vi "HelioScan_3.vi"() -> ()   [LabVIEW 2010]
uses:
  labview_source/controls/update_picture.ctl
  common/xcontrols/XUserDropdown/XUserDropdown/XUserDropdown.xctl
  tools/HelioUpdateMH100803/HelioUpdateMH100803/HelioUpdateMH100803.lvclass
  common/classes/ErrorController/ErrorController/ErrorController.lvclass
  labview_source/type_definitions/clusters/controls_refs.ctl
  components/DAQ/GenericDAQ/GenericDAQ/GenericDAQ.lvclass
  components/ImageAssembler/GenericImageAssembler/GenericImageAssembler/GenericImageAssembler.lvclass
  components/DataCollection/GenericDataCollection/GenericDataCollection/GenericDataCollection.lvclass
  components/Display/GenericDisplay/GenericDisplay/GenericDisplay.lvclass
  components/Analyser/GenericAnalyser/GenericAnalyser/GenericAnalyser.lvclass
  components/ImagingMode/GenericImagingMode/GenericImagingMode/GenericImagingMode.lvclass
  components/Instrument/GenericInstrument/GenericInstrument/GenericInstrument.lvclass
  components/ScanHead/GenericScanHead/GenericScanHead/GenericScanHead.lvclass
  components/Stimulator/GenericStimulator/GenericStimulator/GenericStimulator.lvclass
  components/ExperimentController/GenericExperimentController/GenericExperimentController/GenericExperimentController.lvclass
  components/Stage/GenericStage/GenericStage/GenericStage.lvclass
  <vilib>/Utility/miscctls.llb/LVPointTypeDef.ctl
  components/DataCollection/GenericDataCollection/GenericDataCollection/trigger_enum.ctl
  common/classes/GenericComponent/GenericComponent/GenericComponent.lvclass
  <vilib>/Platform/browser.llb/Open URL in Default Browser (string).vi
  common/classes/ErrorController/ErrorController/class_data.vi
panel:
  out "saving message":string
  out "progress slider":u8(slide) caption="slider" scale=0.0..11.0
  in  "button:start_experiment":bool
  in  "button:start_single_sweep":bool
  in  "button:start_focus":bool
  in  "user":string(xcontrol)
  out "update icon":T1
  in  "file base name":string
  in  "data folder path":path
  in  "notebook":string caption="Notebook"
  in  "exit_button":bool
  in  "objective":string(combo)
  in  "save button":bool
  in  "settings tab":T2(tab)
  in  "imaging mode":string(combo)
  in  "experimental protocol":string(combo)
  in  "stimulator enabled?":bool
  in  "button: task manager":bool
  out "error handler":bool caption="error controller"
  out "experiment controller":bool
  out "imaging mode":bool
  out "scan head":bool
  out "DAQ":bool
  out "image assembler":bool
  out "data collection":bool
  out "display":bool
  out "analyser":bool
  out "stage":bool
  out "stimulator":bool
  out "instrument":bool
  out "Message":string="No Error"
  in  "title":bool caption="HelioScan 3.10.0"
  # "Note: stimulator only works in \"single sweep mode\" and \"experiment mode\"!"
  # "Loaded"
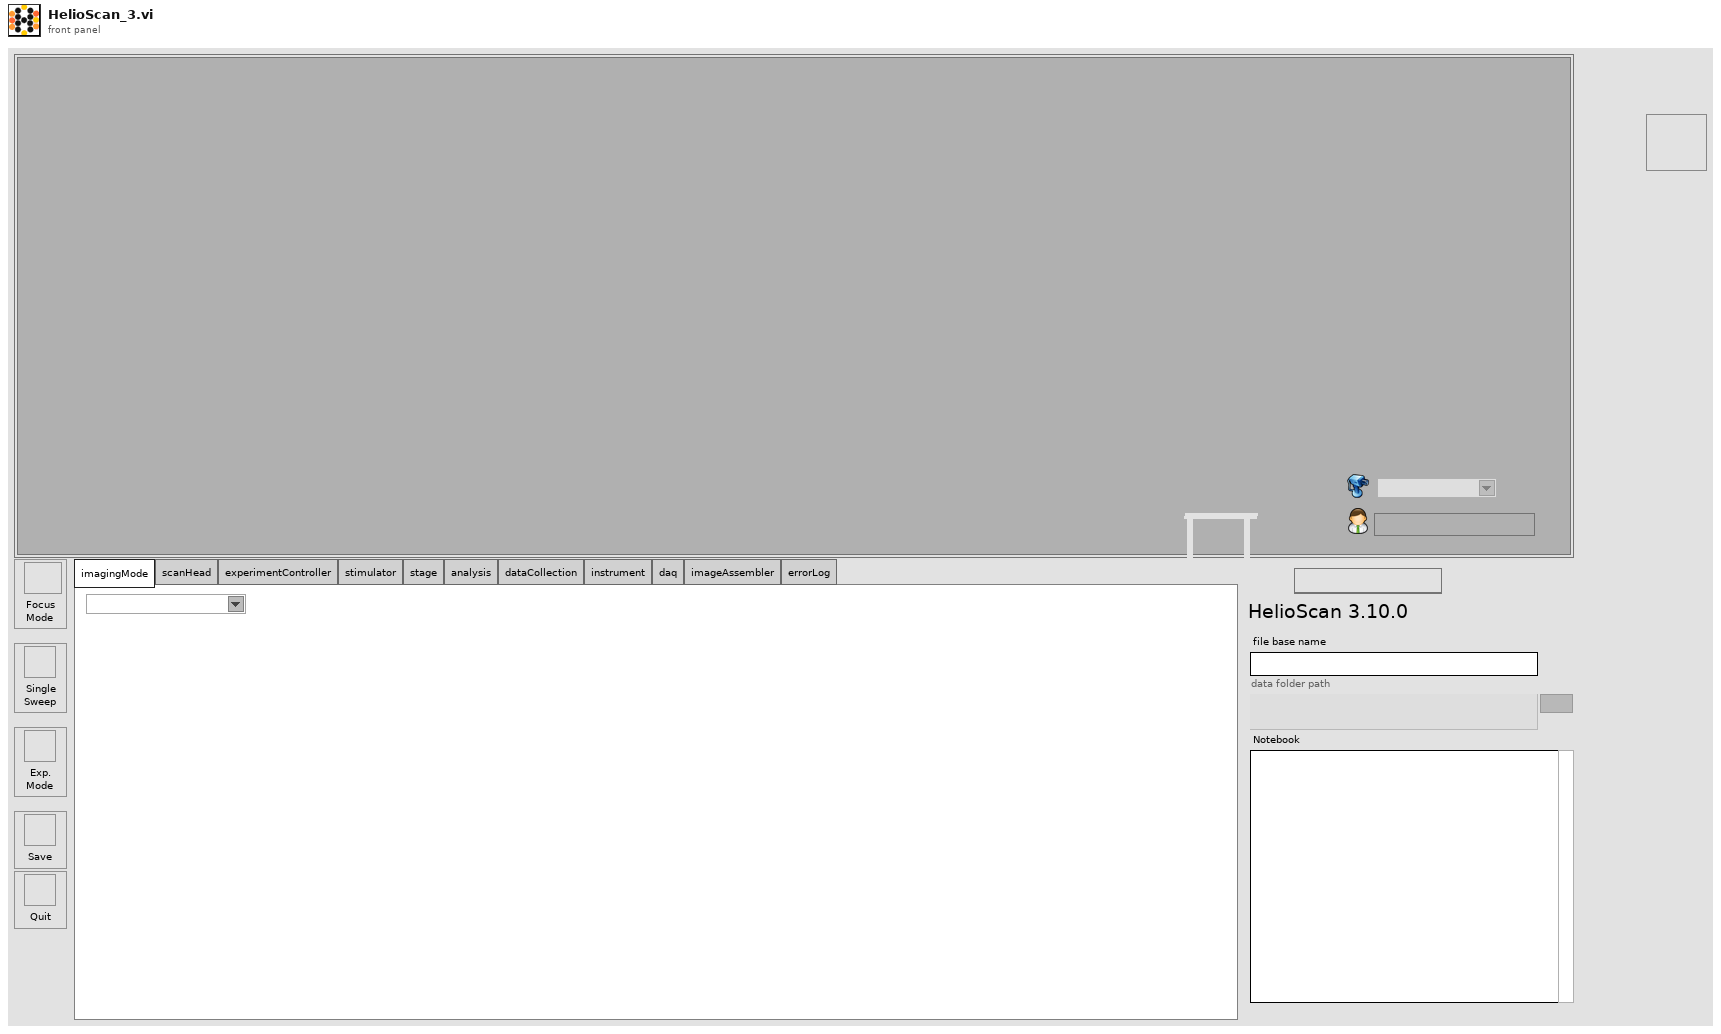
[diagram p1: front panel]
types:
  T1 = typedef "HelioUpdateMH100803.lvclass/update_picture.ctl" = u16
  T2 = enum32{"imagingMode", "scanHead", "experimentController", "stimulator", "stage", "analysis", "dataCollection", "instrument", "daq", "imageAssembler", "errorLog"}
  T3 = typedef "controls_refs.ctl" = cluster{"buttons":cluster{"start_focus":refnum<vi>, "start_single_sweep":refnum<vi>, "start_experiment":refnum<vi>, "save":refnum<vi>, "exit":refnum<vi>}, "tabs":cluster{"main":refnum<vi>, "settings":refnum<vi>}, "subpanels":cluster{"imagingMode":refnum<vi>, "scanHead":refnum<vi>, "display":refnum<vi>, "experimentController":refnum<vi>, "instrument":refnum<vi>, "stage":refnum<vi>, "stimulator":refnum<vi>, "dataCollection":refnum<vi>, "analyser":refnum<vi>, "daq":refnum<vi>, "imageAssembler":refnum<vi>}, "drop-downs":cluster{"imagingMode":refnum<vi>, "experimentalController":refnum<vi>, "objective":refnum<vi>}, "status lights":cluster{"experimentController":refnum<vi>, "imagingMode":refnum<vi>, "scanHead":refnum<vi>, "daq":refnum<vi>, "imageAssembler":refnum<vi>, "dataCollection":refnum<vi>, "display":refnum<vi>, "analyser":refnum<vi>, "stage":refnum<vi>, "stimulator":refnum<vi>, "instrument":refnum<vi>}, "message":refnum<vi>, "stimulator enabled?":refnum<vi>, "saving":cluster{"data folder path":refnum<vi>, "file base name":refnum<vi>, "notebook":refnum<vi>}, "progress bar":refnum<vi>, "update icon":refnum<vi>, "title":refnum<vi>, "main vi":refnum<vi>, "user":refnum<vi>}
  T4 = typedef "LVPointTypeDef.ctl" = cluster{"Horizontal":i16, "Vertical":i16}
  T5 = typedef "GenericDataCollection.lvclass/trigger_enum.ctl" = enum16{"NULL", "save", "reset"}
  T6 = enum32{"Invalid", "Standard", "Closed", "Hidden", "Minimized", "Maximized"}
  T7 = enum8{"Enabled", "Disabled", "Disabled and Grayed Out"}
  T8 = enum16{"focus mode", "single sweep mode", "experiment mode"}
  T9 = typedef "main_trigger_enum.ctl" = enum16{"NULL", "initialise", "terminate", "start", "stop", "change objective", "change experimentController", "change imagingMode", "save notebook", "started saving", "finished saving", "expCtr ready", "expCtr missing", "imgMd ready", "imgMd missing", "scanHd ready", "scanHd missing", "DAQ ready", "DAQ missing", "imgAsm ready", "imgAsm missing", "dataColl ready", "dataColl missing", "display ready", "display missing", "analysr ready", "analysr missing", "instrmnt ready", "instrmnt missing", "stimltr ready", "stimltr missing", "stage ready", "stage missing"}
  T10 = typedef "run_mode_enum.ctl" = enum16{"focus mode", "single sweep mode", "experiment mode"}
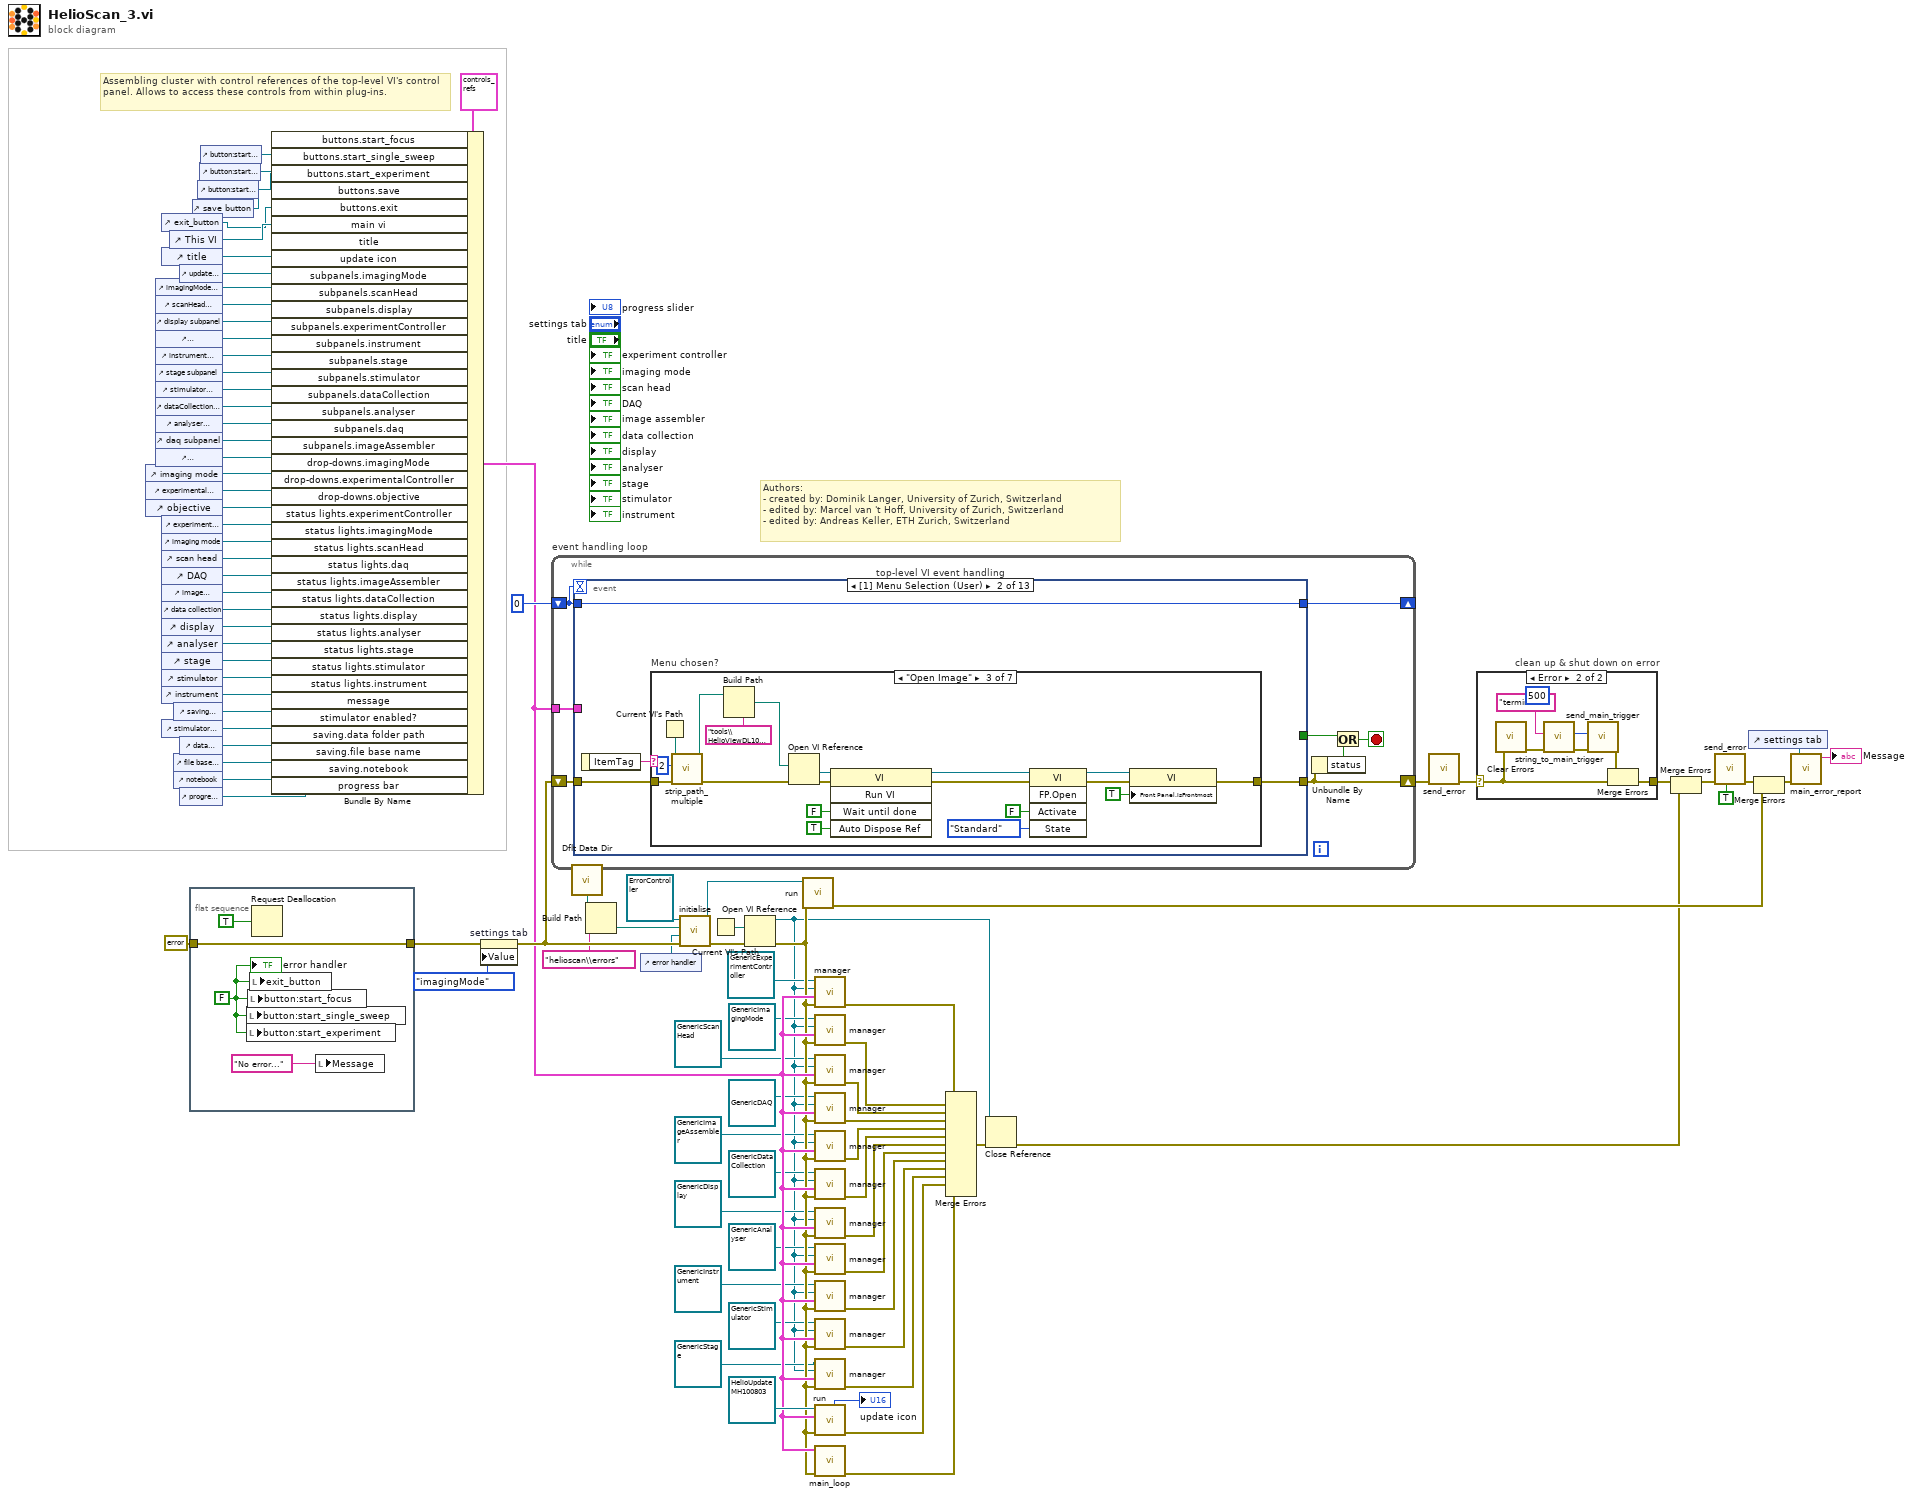
[diagram p0: block diagram]
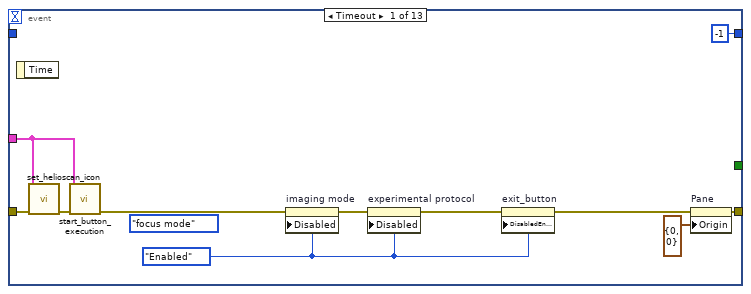
[diagram p3: hidden frame]
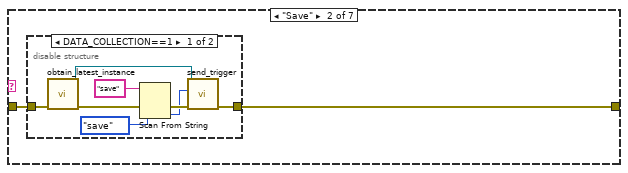
[diagram p5: hidden frame]
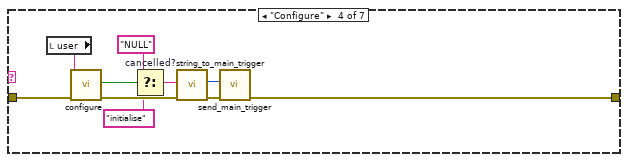
[diagram p7: hidden frame]
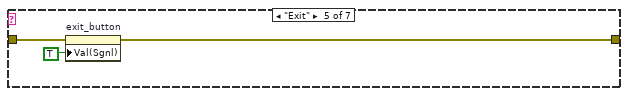
[diagram p8: hidden frame]
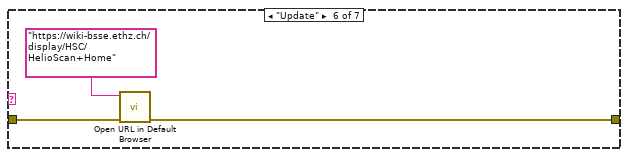
[diagram p9: hidden frame]
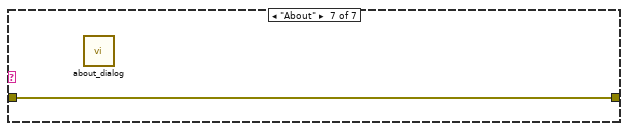
[diagram p10: hidden frame]
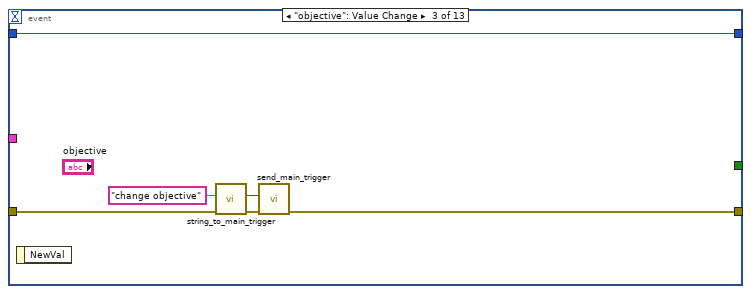
[diagram p11: hidden frame]
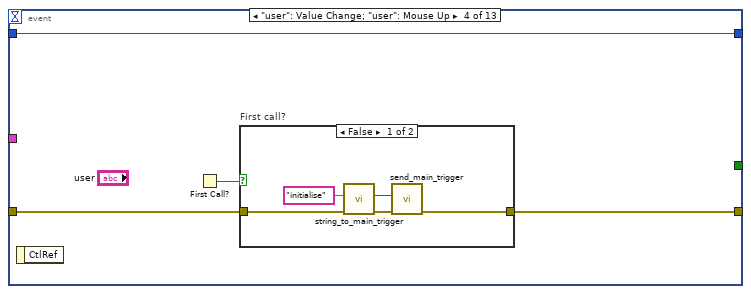
[diagram p12: hidden frame]
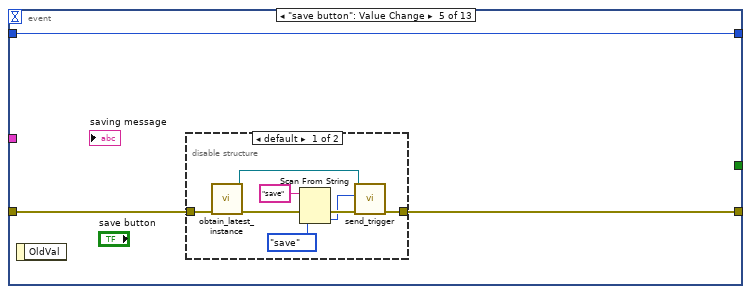
[diagram p14: hidden frame]
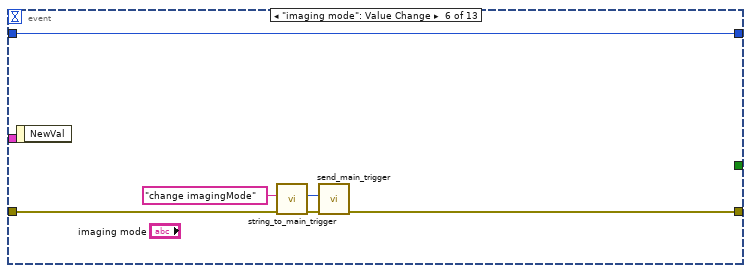
[diagram p16: hidden frame]
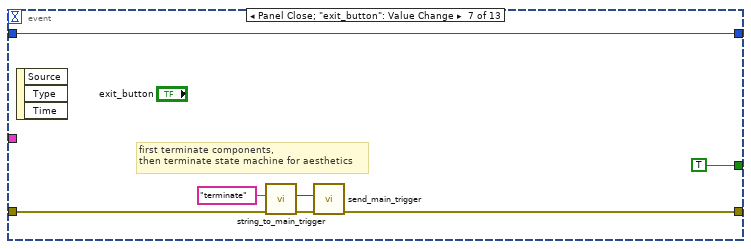
[diagram p17: hidden frame]
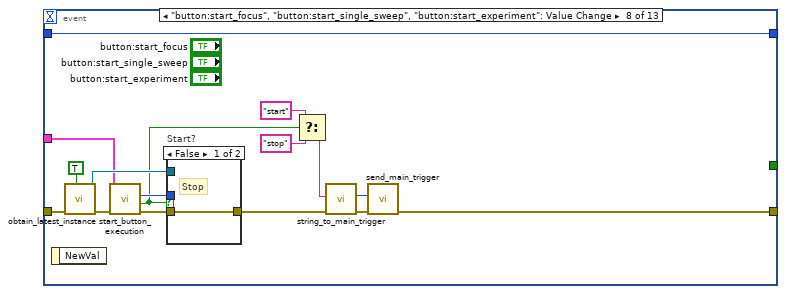
[diagram p18: hidden frame]
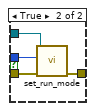
[diagram p19: hidden frame]
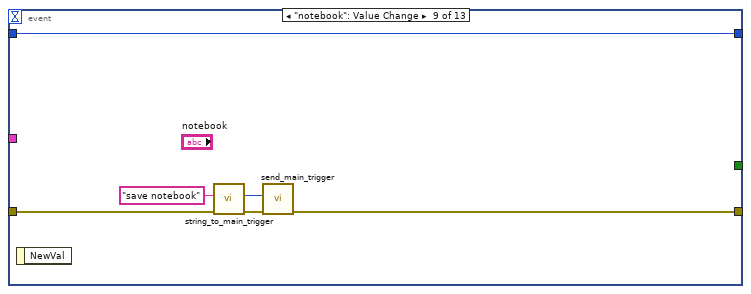
[diagram p20: hidden frame]
diagram:
  # "Authors: \n- created by: Dominik Langer, University of Zurich, Switzerland\n- edited by: Marcel van 't Hoff, University of Zurich, Switzerland\n- edited by: Andreas Keller, ETH Zurich, Switzerland"
  # "Assembling cluster with control references of the top-level VI's control panel. Allows to access these controls from within plug-ins."
  n1 = control-ref of="imaging mode"() -> (w83:refnum<vi>)
  n2 = control-ref of="experimental protocol"() -> (w84:refnum<vi>)
  n3 = control-ref of="objective"() -> (w69:refnum<vi>)
  n4 = control-ref of="imagingMode subpanel"() -> (w63:refnum<vi>)
  n5 = control-ref of="scanHead subpanel"() -> (w94:refnum<vi>)
  n6 = control-ref of="display subpanel"() -> (w90:refnum<vi>)
  n7 = control-ref of="experimentController subpanel"() -> (w91:refnum<vi>)
  n8 = control-ref of="instrument subpanel"() -> (w89:refnum<vi>)
  n9 = control-ref of="stage subpanel"() -> (w87:refnum<vi>)
  n10 = control-ref of="stimulator subpanel"() -> (w86:refnum<vi>)
  n11 = control-ref of="dataCollection subpanel"() -> (w85:refnum<vi>)
  n12 = control-ref of="analyser subpanel"() -> (w82:refnum<vi>)
  n13 = control-ref of="daq subpanel"() -> (w61:refnum<vi>)
  n14 = control-ref of="imageAssembler subpanel"() -> (w62:refnum<vi>)
  n15 = control-ref of="exit_button"() -> (w1:refnum<vi>)
  n16 = control-ref of="title"() -> (w44:refnum<vi>)
  n17 = control-ref of="experiment controller"() -> (w73:refnum<vi>)
  n18 = control-ref of="imaging mode"() -> (w72:refnum<vi>)
  n19 = control-ref of="scan head"() -> (w76:refnum<vi>)
  n20 = control-ref of="DAQ"() -> (w75:refnum<vi>)
  n21 = control-ref of="image assembler"() -> (w74:refnum<vi>)
  n22 = control-ref of="data collection"() -> (w71:refnum<vi>)
  n23 = control-ref of="display"() -> (w77:refnum<vi>)
  n24 = control-ref of="analyser"() -> (w78:refnum<vi>)
  n25 = control-ref of="stage"() -> (w81:refnum<vi>)
  n26 = control-ref of="stimulator"() -> (w80:refnum<vi>)
  n27 = control-ref of="instrument"() -> (w70:refnum<vi>)
  n28 = control-ref of="stimulator enabled?"() -> (w67:refnum<vi>)
  n29 = control-ref of="This VI"() -> (w41:refnum<vi>)
  n30 = control-ref of="saving message"() -> (w45:refnum<vi>)
  n31 = control-ref of="file base name"() -> (w65:refnum<vi>)
  n32 = control-ref of="notebook"() -> (w64:refnum<vi>)
  n33 = control-ref of="update icon"() -> (w43:refnum<vi>)
  n34 = control-ref of="data folder path"() -> (w66:refnum<vi>)
  n35 = control-ref of="progress bar"() -> (w49:refnum<vi>)
  n36 = flat-sequence {
    tunnel: errorcluster {"status"=FALSE, "code"=0, "source"=""} ("error in (no error)") -> [w98]
    tunnel: [w98] -> w7
    frame #0 {
      w95 = FALSE
      n37 = local write "button:start_single_sweep"(w95) -> ()
      n38 = local write "button:start_experiment"(w95) -> ()
      n39 = local write "button:start_focus"(w95) -> ()
      n40 = local write "exit_button"(w95) -> ()
      n41 = Request Deallocation(TRUE ("flag")) -> ()
      n42 = local write "Message"("No error...") -> ()
      "error handler" <- w95
    }
  }
  n43 = control-ref of="save button"() -> (w2:refnum<vi>)
  n44 = control-ref of="button:start_experiment"() -> (w3:refnum<vi>)
  n45 = control-ref of="button:start_single_sweep"() -> (w4:refnum<vi>)
  n46 = control-ref of="button:start_focus"() -> (w5:refnum<vi>)
  n47 = Bundle By Name(cluster=T3 {"buttons"={"start_focus"=refnum, "start_single_sweep"=refnum, "start_experiment"=refnum, "save"=refnum, "exit"=refnum}, "tabs"={"main"=refnum, "settings"=refnum}, "subpanels"={"imagingMode"=refnum, "scanHead"=refnum, "display"=refnum, "experimentController"=refnum, "instrument"=refnum, "stage"=refnum, "stimulator"=refnum, "dataCollection"=refnum, "analyser"=refnum, "daq"=refnum, "imageAssembler"=refnum}, "drop-downs"={"imagingMode"=refnum, "experimentalController"=refnum, "objective"=refnum}, "status lights"={"experimentController"=refnum, "imagingMode"=refnum, "scanHead"=refnum, "daq"=refnum, "imageAssembler"=refnum, "dataCollection"=refnum, "display"=refnum, "analyser"=refnum, "stage"=refnum, "stimulator"=refnum, "instrument"=refnum}, "message"=refnum, "stimulator enabled?"=refnum, "saving"={"data folder path"=refnum, "file base name"=refnum, "notebook"=refnum}, "progress bar"=refnum, "update icon"=refnum, "title"=refnum, "main vi"=refnum, "user"=refnum} ("control references"), "buttons.start_focus"=w5, "buttons.start_single_sweep"=w4, "buttons.start_experiment"=w3, "buttons.save"=w2, "buttons.exit"=w1, "main vi"=w41, "title"=w44, "update icon"=w43, "subpanels.imagingMode"=w63, "subpanels.scanHead"=w94, "subpanels.display"=w90, "subpanels.experimentController"=w91, "subpanels.instrument"=w89, "subpanels.stage"=w87, "subpanels.stimulator"=w86, "subpanels.dataCollection"=w85, "subpanels.analyser"=w82, "subpanels.daq"=w61, "subpanels.imageAssembler"=w62, "drop-downs.imagingMode"=w83, "drop-downs.experimentalController"=w84, "drop-downs.objective"=w69, "status lights.experimentController"=w73, "status lights.imagingMode"=w72, "status lights.scanHead"=w76, "status lights.daq"=w75, "status lights.imageAssembler"=w74, "status lights.dataCollection"=w71, "status lights.display"=w77, "status lights.analyser"=w78, "status lights.stage"=w81, "status lights.stimulator"=w80, "status lights.instrument"=w70, "message"=w45, "stimulator enabled?"=w67, "saving.data folder path"=w66, "saving.file base name"=w65, "saving.notebook"=w64, "progress bar"=w49) -> (w23:T3)
  n48 = property on="settings tab" class="TabCtl (strict)"(error in=w7, "Value"=T2."imagingMode" ("settings tab")) -> (error out=w35:errorcluster)  [unwired: 1 in, 1 out]
  n49 = while "event handling loop" {
    shift-right: [w104] -> _
    shift-left: 0 -> [w105]
    tunnel: w23 -> [w103]
    shift-right: [w102] -> w38
    shift-left: w35 -> [w106]
    stop <- w99 stop-if-true
    n50 = event "top-level VI event handling" shown="[1] Menu Selection (User)" {
      selector: _ -> [_ _ _ _ _ _ _ _ _ _ _ _ _]
      dyn-events: _ -> [_ _ _ _ _ _ _ _ _ _ _ _ _]
      timeout: w105 -> [_ _ _ _ _ _ _ _ _ _ _ _ _]
      tunnel: [_ _ _ _ _ _ TRUE _ _ _ _ _ _] -> w101
      tunnel: [w115 w118 w174 w178 w187 w202 w208 w212 w236 w242 w251 w262 w268] -> w102
      tunnel: w106 -> [w111 w119 w173 w176 w186 w201 w204 w216 w235 w243 w256 w259 w279]
      tunnel: [-1 w121 w175 w179 w188 w203 w210 w226 w237 w245 w257 w263 w280] -> w104
      tunnel: w105 -> [_ w121 w175 w179 w188 w203 w210 w226 w237 w245 w257 w263 w280]
      tunnel: w103 -> [w109 _ _ _ _ _ _ w213 _ _ _ _ _]
      event Timeout {
        w112 = T7."Enabled" ("Disabled")
        (unwired) T8."focus mode" ("Value (Signaling)")
        n51 = event-data() -> ()  [unwired: 2 out]
        n52 = call "set_helioscan_icon.vi"("error in (no error)"=w111, "reference cluster in"=w109) -> ("error out"=w110:errorcluster)  [unwired: 9 in]
        n53 = call "start_button_execution.vi"("error in (no error)"=w110, "control references"=w109) -> ("error out"=w108:errorcluster)  [unwired: 7 in, 2 out]
        n54 = property on="imaging mode" class="CmbBox"(error in=w108, "Disabled"=w112) -> (error out=w116:errorcluster)  [unwired: 1 in, 1 out]
        n55 = property on="experimental protocol" class="CmbBox"(error in=w116, "Disabled"=w112) -> (error out=w113:errorcluster)  [unwired: 1 in, 1 out]
        n56 = property on="exit_button" class="Bool (strict)"(error in=w113, "DisabledEnum"=w112) -> (error out=w107:errorcluster)  [unwired: 1 in, 1 out]
        n57 = property on="Pane" class="Pane"(error in=w107, "Origin"=T4 {"Horizontal"=0, "Vertical"=0}) -> (error out=w115:errorcluster)  [unwired: 1 in, 1 out]
      }
      event Menu Selection (User) {
        n58 = event-data() -> ("ItemTag"=w120:string)  [unwired: 1 out]
        n59 = case "Menu chosen?" shown="\"Open Image\"" w120 {
          tunnel: w119 -> [w122 w124 w149 w162 w165 w168 w169]
          tunnel: [w122 w123 w135 w160 w163 w167 w169] -> w118
          frame Default {
          }
          frame "Save" {
            n60 = disable-structure shown="DATA_COLLECTION==1" {
              disable-tunnel: w124 -> [w131 w133]
              disable-tunnel: [w132 w133] -> w123
              frame condition #0 (active) {
                n61 = call "obtain_latest_instance.vi"("error in (no error)"=w131) -> ("error out"=w128:errorcluster, "GenericDataCollection out"=w130:refnum<class "GenericDataCollection.lvclass">)  [unwired: 1 in, 8 out]
                n62 = Scan From String(input string="save", error in=w128, default 1=trigger_enum."save" ("trigger")) -> (error out=w127:errorcluster, output 1=w126:T5)  [unwired: 2 in, 2 out]
                n63 = call-dynamic "send_trigger.vi"("error in (no error)"=w127, "trigger"=w126, "GenericDataCollection in"=w130) -> ("error out"=w132:errorcluster)  [unwired: 8 out]
              }
              frame condition #1 {
              }
            }
          }
          frame "Open Image" {
            n64 = Current VI's Path() -> (path=w150:path)
            n65 = call "strip_path_multiple.vi"("error in (no error)"=w149, "number of strips"=2, "path in"=w150) -> ("error out"=w148:errorcluster, "path out"=w144:path)  [unwired: 7 in]
            n66 = Build Path(base path=w144, name or relative path="tools\\HelioViewDL100122\\HelioView.vi") -> (appended path=w142:path)
            n67 = Open VI Reference(vi path=w142, error in (no error)=w148) -> (vi reference=w152:refnum<vi>, error out=w151:errorcluster)  [unwired: 4 in]
            n68 = invoke class="VI" method="Run VI"(reference=w152, error in=w151, "Wait until done"=FALSE ("Wait Until Done"), "Auto Dispose Ref"=TRUE ("Auto Dispose Reference")) -> (reference out=w138:refnum<vi>, error out=w141:errorcluster)  [unwired: 1 in, 3 out]
            n69 = invoke class="VI" method="FP.Open"(reference=w138, error in=w141, "Activate"=FALSE ("Activate?"), "State"=T6."Standard") -> (reference out=w134:refnum<vi>, error out=w136:errorcluster)  [unwired: 1 in, 3 out]
            n70 = property class="VI"(reference=w134, error in=w136, "Front Panel.IsFrontmost"=TRUE ("Front Panel Window:Is Frontmost")) -> (error out=w135:errorcluster)  [unwired: 1 out]
          }
          frame "Configure" {
            n71 = local read "user"() -> (w161:string)
            n72 = call "configure.vi"("error in (no error)"=w162, "user"=w161) -> ("error out"=w158:errorcluster, "cancelled?"=w159:bool)  [unwired: 1 in, 7 out]
            n73 = Select "cancelled?"(t="NULL", s=w159, f="initialise") -> (s? t:f=w154:string)
            n74 = call "string_to_main_trigger.vi"("error in (no error)"=w158, "trigger string"=w154) -> ("error out"=w157:errorcluster, "main trigger"=w153:T9)  [unwired: 8 in]
            n75 = call "send_main_trigger.vi"("error in (no error)"=w157, "trigger"=w153) -> ("error out"=w160:errorcluster)  [unwired: 9 in]
          }
          frame "Exit" {
            n76 = property on="exit_button" class="Bool (strict)"(error in=w165, "Val(Sgnl)"=TRUE) -> (error out=w163:errorcluster)  [unwired: 1 in, 1 out]
          }
          frame "Update" {
            n77 = call-poly <vilib>:"Open URL in Default Browser.vi"("error in (no error)"=w168, "URL"="https://wiki-bsse.ethz.ch/display/HSC/HelioScan+Home") -> ("error out"=w167:errorcluster)  [unwired: 4 in, 1 out]
          }
          frame "About" {
            n78 = call "about_dialog.vi"() -> ()  [unwired: 1 out]
          }
        }
      }
      event "objective": Value Change {
        n79 = event-data() -> ()  [unwired: 2 out]
        n80 = call "string_to_main_trigger.vi"("error in (no error)"=w173, "trigger string"="change objective") -> ("error out"=w172:errorcluster, "main trigger"=w171:T9)  [unwired: 8 in]
        n81 = call "send_main_trigger.vi"("error in (no error)"=w172, "trigger"=w171) -> ("error out"=w174:errorcluster)  [unwired: 9 in]
      }
      event "user": Value Change; "user": Mouse Up {
        n82 = event-data() -> ()  [unwired: 2 out]
        n83 = First Call?() -> (First Call?: T/F=w177:bool)
        n84 = case "First call?" shown="False" w177 {
          tunnel: [w184 w185] -> w178
          tunnel: w176 -> [w183 w185]
          frame False {
            n85 = call "string_to_main_trigger.vi"("error in (no error)"=w183, "trigger string"="initialise") -> ("error out"=w182:errorcluster, "main trigger"=w181:T9)  [unwired: 8 in]
            n86 = call "send_main_trigger.vi"("error in (no error)"=w182, "trigger"=w181) -> ("error out"=w184:errorcluster)  [unwired: 9 in]
          }
          frame True {
          }
        }
      }
      event "save button": Value Change {
        n87 = event-data() -> ()  [unwired: 2 out]
        n88 = disable-structure shown="default" {
          disable-tunnel: [w196 w197] -> w187
          disable-tunnel: w186 -> [w195 w197]
          frame condition #0 (active) {
            n89 = call "obtain_latest_instance.vi"("error in (no error)"=w195) -> ("error out"=w193:errorcluster, "GenericDataCollection out"=w194:refnum<class "GenericDataCollection.lvclass">)  [unwired: 1 in, 8 out]
            n90 = Scan From String(input string="save", error in=w193, default 1=trigger_enum."save" ("trigger")) -> (error out=w192:errorcluster, output 1=w190:T5)  [unwired: 2 in, 2 out]
            n91 = call-dynamic "send_trigger.vi"("error in (no error)"=w192, "trigger"=w190, "GenericDataCollection in"=w194) -> ("error out"=w196:errorcluster)  [unwired: 8 out]
          }
          frame condition #1 {
          }
        }
      }
      event "imaging mode": Value Change {
        n92 = event-data() -> ()  [unwired: 2 out]
        n93 = call "string_to_main_trigger.vi"("error in (no error)"=w201, "trigger string"="change imagingMode") -> ("error out"=w200:errorcluster, "main trigger"=w199:T9)  [unwired: 8 in]
        n94 = call "send_main_trigger.vi"("error in (no error)"=w200, "trigger"=w199) -> ("error out"=w202:errorcluster)  [unwired: 9 in]
      }
      event Panel Close; "exit_button": Value Change {
        # "first terminate components, \nthen terminate state machine for aesthetics"
        n95 = event-data() -> ()  [unwired: 4 out]
        n96 = call "string_to_main_trigger.vi"("error in (no error)"=w204, "trigger string"="terminate") -> ("error out"=w207:errorcluster, "main trigger"=w206:T9)  [unwired: 8 in]
        n97 = call "send_main_trigger.vi"("error in (no error)"=w207, "trigger"=w206) -> ("error out"=w208:errorcluster)  [unwired: 9 in]
      }
      event "button:start_focus", "button:start_single_sweep", "button:start_experiment": Value Change {
        n98 = event-data() -> ()  [unwired: 2 out]
        n99 = call "obtain_latest_instance.vi"("quick, but maybe outdated?"=TRUE, "error in (no error)"=w216) -> ("error out"=w215:errorcluster, "GenericScanMode out"=w225:refnum<class "GenericImagingMode.lvclass">)  [unwired: 8 out]
        n100 = call "start_button_execution.vi"("error in (no error)"=w215, "control references"=w213) -> ("error out"=w214:errorcluster, "start?"=w211:bool, "mode"=w217:T10)  [unwired: 7 in]
        n101 = case "Start?" shown="False" w211 {
          tunnel: w225 -> [_ w231]
          tunnel: [w227 w230] -> w218
          tunnel: w217 -> [_ w229]
          tunnel: w214 -> [w227 w228]
          frame False {
            # "Stop"
          }
          frame True {
            n102 = call-dynamic "set_run_mode.vi"("error in (no error)"=w228, "run mode"=w229, "GenericPlugin in"=w231) -> ("error out"=w230:errorcluster)  [unwired: 8 out]
          }
        }
        n103 = Select(t="start" ("trigger string"), s=w211, f="stop") -> (s? t:f=w220:string)
        n104 = call "string_to_main_trigger.vi"("error in (no error)"=w218, "trigger string"=w220) -> ("error out"=w222:errorcluster, "main trigger"=w223:T9)  [unwired: 8 in]
        n105 = call "send_main_trigger.vi"("error in (no error)"=w222, "trigger"=w223) -> ("error out"=w212:errorcluster)  [unwired: 9 in]
      }
      event "notebook": Value Change {
        n106 = event-data() -> ()  [unwired: 2 out]
        n107 = call "string_to_main_trigger.vi"("error in (no error)"=w235, "trigger string"="save notebook") -> ("error out"=w234:errorcluster, "main trigger"=w233:T9)  [unwired: 8 in]
        n108 = call "send_main_trigger.vi"("error in (no error)"=w234, "trigger"=w233) -> ("error out"=w236:errorcluster)  [unwired: 9 in]
      }
      event "file base name", "data folder path": Value Change {
        n109 = event-data() -> ()  [unwired: 2 out]
        n110 = call-dynamic "set_data_folder_path.vi"("error in (no error)"=w243, "data folder path"="data folder path", "GenericComponent in"=refnum<class "GenericComponent.lvclass"> refnum ("GenericComponent.lvclass")) -> ("error out"=w244:errorcluster, "GenericComponent out"=w239:refnum<class "GenericComponent.lvclass">)  [unwired: 7 out]
        n111 = call-dynamic "set_file_name_base.vi"("error in (no error)"=w244, "file name base"="file base name", "GenericComponent in"=w239) -> ("error out"=w242:errorcluster)  [unwired: 8 out]
      }
      event "stimulator enabled?": Value Change {
        n112 = event-data() -> ("NewVal"=w246:bool)  [unwired: 1 out]
        n113 = Select(t=T7."Enabled" ("Disabled"), s=w246, f=T7."Disabled and Grayed Out") -> (s? t:f=w254:T7)
        n114 = property on="stimulator\nsubpanel" class="SubPnl"(error in=w256, "DisabledEnum"=w254) -> (error out=w252:errorcluster)  [unwired: 1 in, 1 out]
        n115 = call "checkout.vi"("error in (no error)"=w252) -> ("error out"=w249:errorcluster, "GenericStimulator out"=w250:refnum<class "GenericStimulator.lvclass">)  [unwired: 9 in]
        n116 = call-dynamic "set_enabled_state.vi"("error in (no error)"=w249, "enabled?"=w246, "GenericStimulator in"=w250) -> ("error out"=w248:errorcluster, "GenericStimulator out"=w247:refnum<class "GenericStimulator.lvclass">)  [unwired: 7 in]
        n117 = call-dynamic "checkin.vi"("error in (no error)"=w248, "GenericStimulator in"=w247) -> ("error out"=w251:errorcluster)  [unwired: 8 in, 1 out]
      }
      event "experimental protocol": Value Change {
        n118 = event-data() -> ()  [unwired: 2 out]
        n119 = call "string_to_main_trigger.vi"("error in (no error)"=w259, "trigger string"="change experimentController") -> ("error out"=w260:errorcluster, "main trigger"=w261:T9)  [unwired: 8 in]
        n120 = call "send_main_trigger.vi"("error in (no error)"=w260, "trigger"=w261) -> ("error out"=w262:errorcluster)  [unwired: 9 in]
      }
      event "button: task manager": Value Change {
        n121 = event-data() -> ()  [unwired: 2 out]
        n122 = Current VI's Path() -> (path=w278:path)
        n123 = call "strip_path_multiple.vi"("error in (no error)"=w279, "number of strips"=2, "path in"=w278) -> ("error out"=w273:errorcluster, "path out"=w276:path)  [unwired: 7 in]
        n124 = Build Path(base path=w276, name or relative path="common\\utilities\\task_manager.vi") -> (appended path=w274:path)
        n125 = Open VI Reference(vi path=w274, error in (no error)=w273) -> (vi reference=w272:refnum<vi>, error out=w271:errorcluster)  [unwired: 4 in]
        n126 = invoke class="VI" method="Run VI"(reference=w272, error in=w271, "Wait until done"=FALSE ("Wait Until Done"), "Auto Dispose Ref"=TRUE ("Auto Dispose Reference")) -> (reference out=w270:refnum<vi>, error out=w269:errorcluster)  [unwired: 1 in, 3 out]
        n127 = invoke class="VI" method="FP.Open"(reference=w270, error in=w269, "Activate"=TRUE ("Activate?"), "State"=T6."Standard") -> (error out=w268:errorcluster)  [unwired: 1 in, 4 out]
      }
    }
    n128 = Unbundle By Name(w102) -> ("status"=w100:bool)
    n129 = Or(x=w101, y=w100) -> (x .or. y?=w99:bool)
  }
  n130 = call <vilib>:"Dflt Data Dir.vi"() -> ("App:Default Data Directory"=w26:path)
  n131 = Build Path(base path=w26, name or relative path="helioscan\\errors") -> (appended path=w24:path)
  n132 = control-ref of="error handler"() -> (w27:refnum<vi>)
  n133 = call-dynamic "initialise.vi"("error in (no error)"=w35, "error boolean"=w27, "error file store path"=w24, "ErrorController in"=refnum<class "ErrorController.lvclass"> refnum) -> ("error out"=w34:errorcluster, "ErrorController out"=w33:refnum<class "ErrorController.lvclass">)  [unwired: 6 in]
  n134 = Current VI's Path() -> (path=w88:path)
  n135 = Open VI Reference(vi path=w88, error in (no error)=w34) -> (vi reference=w10:refnum<vi>, error out=w22:errorcluster)  [unwired: 1 in, 3 out]
  n136 = call "run.vi"("error in (no error)"=w22, "ErrorController in"=w33) -> ("error out"=w32:errorcluster)  [unwired: 8 in, 1 out]
  n137 = call-dynamic "manager.vi"("error in (no error)"=w22, "control references"=w23, "top-level VI ref in"=w10, "GenericToplevelComponent in"=refnum<class "GenericExperimentController.lvclass"> refnum ("GenericExperimentController.lvclass")) -> ("error out"=w50:errorcluster)  [unwired: 5 in, 2 out]
  n138 = call-dynamic "manager.vi"("error in (no error)"=w22, "control references"=w23, "top-level VI ref in"=w10, "GenericToplevelComponent in"=refnum<class "GenericImagingMode.lvclass"> refnum ("GenericImagingMode.lvclass")) -> ("error out"=w53:errorcluster)  [unwired: 5 in, 2 out]
  n139 = call-dynamic "manager.vi"("error in (no error)"=w22, "control references"=w23, "top-level VI ref in"=w10, "GenericToplevelComponent in"=refnum<class "GenericScanHead.lvclass"> refnum ("GenericScanHead.lvclass")) -> ("error out"=w52:errorcluster)  [unwired: 5 in, 2 out]
  n140 = call-dynamic "manager.vi"("error in (no error)"=w22, "control references"=w23, "top-level VI ref in"=w10, "GenericToplevelComponent in"=refnum<class "GenericDAQ.lvclass"> refnum ("GenericDAQ.lvclass")) -> ("error out"=w51:errorcluster)  [unwired: 5 in, 2 out]
  n141 = call-dynamic "manager.vi"("error in (no error)"=w22, "control references"=w23, "top-level VI ref in"=w10, "GenericToplevelComponent in"=refnum<class "GenericImageAssembler.lvclass"> refnum ("GenericImageAssembler.lvclass")) -> ("error out"=w60:errorcluster)  [unwired: 5 in, 2 out]
  n142 = call-dynamic "manager.vi"("error in (no error)"=w22, "control references"=w23, "top-level VI ref in"=w10, "GenericToplevelComponent in"=refnum<class "GenericDataCollection.lvclass"> refnum ("GenericDataCollection.lvclass")) -> ("error out"=w59:errorcluster)  [unwired: 5 in, 2 out]
  n143 = call-dynamic "manager.vi"("error in (no error)"=w22, "control references"=w23, "top-level VI ref in"=w10, "GenericToplevelComponent in"=refnum<class "GenericDisplay.lvclass"> refnum ("GenericDisplay.lvclass")) -> ("error out"=w58:errorcluster)  [unwired: 5 in, 2 out]
  n144 = call-dynamic "manager.vi"("error in (no error)"=w22, "control references"=w23, "top-level VI ref in"=w10, "GenericToplevelComponent in"=refnum<class "GenericAnalyser.lvclass"> refnum ("GenericAnalyser.lvclass")) -> ("error out"=w57:errorcluster)  [unwired: 5 in, 2 out]
  n145 = call-dynamic "manager.vi"("error in (no error)"=w22, "control references"=w23, "top-level VI ref in"=w10, "GenericToplevelComponent in"=refnum<class "GenericInstrument.lvclass"> refnum ("GenericInstrument.lvclass")) -> ("error out"=w56:errorcluster)  [unwired: 5 in, 2 out]
  n146 = call-dynamic "manager.vi"("error in (no error)"=w22, "control references"=w23, "top-level VI ref in"=w10, "GenericToplevelComponent in"=refnum<class "GenericStimulator.lvclass"> refnum ("GenericStimulator.lvclass")) -> ("error out"=w55:errorcluster)  [unwired: 5 in, 2 out]
  n147 = call-dynamic "manager.vi"("error in (no error)"=w22, "control references"=w23, "top-level VI ref in"=w10, "GenericToplevelComponent in"=refnum<class "GenericStage.lvclass"> refnum ("GenericStage.lvclass")) -> ("error out"=w54:errorcluster)  [unwired: 5 in, 2 out]
  n148 = call-dynamic "run.vi"("error in (no error)"=w22, "control references"=w23, "HelioUpdateMH100803 in"=refnum<class "HelioUpdateMH100803.lvclass"> refnum) -> ("error out"=w42:errorcluster, "update out"=→"update icon":T1)  [unwired: 6 in, 1 out]
  n149 = call "main_loop.vi"("error in (no error)"=w22, "control references"=w23) -> ("error out"=w9:errorcluster)  [unwired: 9 in]
  n150 = Merge Errors(w50, w53, w52, w51, w60, w59, w58, w57, w56, w55, w54, w42, w9) -> (w68:errorcluster)
  n151 = Close Reference(reference=w10, error in (no error)=w68) -> (error out=w8:errorcluster)
  n152 = call "send_error.vi"("error in (no error)"=w38) -> ("error out"=w30:errorcluster)  [unwired: 10 in]
  n153 = case "clean up & shut down on error" shown="Error" w30 {
    selector: w30 -> [w281 w287]
    tunnel: [w281 w286] -> w28
    frame No Error {
    }
    frame Error {
      (unwired) u32 500 ("milliseconds to wait")
      n154 = call <vilib>:"Clear Errors.vi"("error in (no error)"=w287) -> ("error out"=w285:errorcluster)  [unwired: 6 in]
      n155 = call "string_to_main_trigger.vi"("error in (no error)"=w285, "trigger string"="terminate") -> ("error out"=w284:errorcluster, "main trigger"=w282:T9)  [unwired: 8 in]
      n156 = call "send_main_trigger.vi"("error in (no error)"=w284, "trigger"=w282) -> ("error out"=w288:errorcluster)  [unwired: 9 in]
      n157 = Merge Errors(w288, w287) -> (w286:errorcluster)
    }
  }
  n158 = Merge Errors(w28, w8) -> (w29:errorcluster)
  n159 = call "send_error.vi"("last error? (F)"=TRUE, "error in (no error)"=w29) -> ("error out"=w37:errorcluster)  [unwired: 9 in]
  n160 = control-ref of="settings tab"() -> (w40:refnum<vi>)
  n161 = Merge Errors(w37, w32) -> (w36:errorcluster)
  n162 = call "main_error_report.vi"("error in"=w36, "TabCtl Refnum"=w40) -> ("message"=→"Message":string)  [unwired: 9 in]
